vi "H5Sget_simple_extent_dims.vi"(6 "error in (no error)":errorcluster, 9 "HDF5 Space Ref":T1) -> (0 "error out":errorcluster, 1 "Max Dims":u64[](array[numeric]), 2 "Dims":u64[](array[numeric]), 3 "HDF5 Ref out":T1)   [LabVIEW 2017]
doc: "Retrieves dataspace dimension size and maximum size."
uses:
  <vilib>/UPVI/lvhdf5/library.llb/HDF5 Ref.ctl
  <vilib>/UPVI/lvhdf5/hdf5.dll
panel:
  # "LVHDF5 Toolkit\nCopyright (c) 2005-2013 by Jason D. Sommerville\nCopyright (c) 2014 by UPVI, LLC.\n\nThis use and distribution of this file is governed by the terms found in \nLICENSE.txt distributed with this toolkit and installed at\n <user.lib>\\_lvhdf5\\LICENSE.txt"
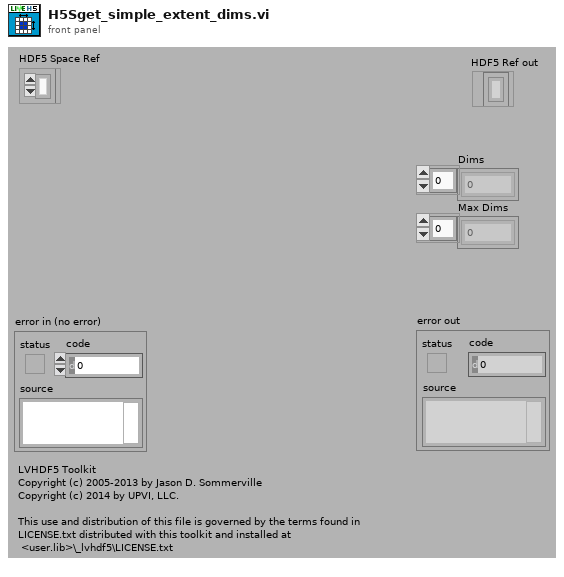
[diagram p1: front panel]
types:
  T1 = typedef "HDF5 Ref.ctl" = refnum<k1>
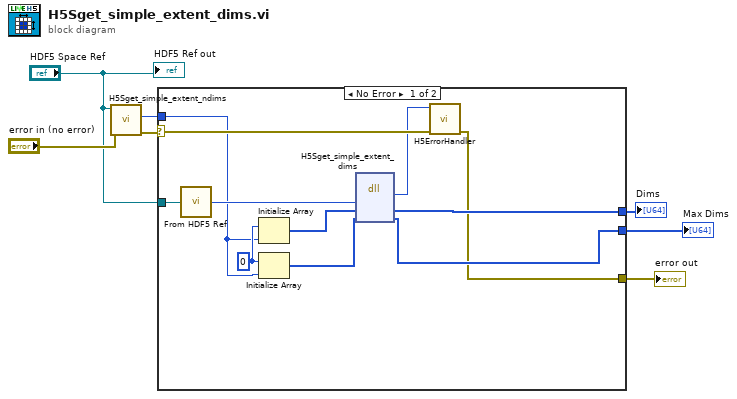
[diagram p0: block diagram]
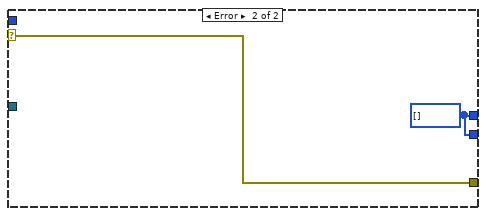
[diagram p2: hidden frame]
diagram:
  n1 = call <vilib>:"H5Sget_simple_extent_ndims.vi"("error in (no error)"="error in (no error)", "HDF5 Space Ref"="HDF5 Space Ref") -> ("error out"=w5:errorcluster, "Rank"=w3:i32)  [unwired: 5 in, 1 out]
  n2 = case shown="No Error" w5 {
    selector: w5 -> [w18 w20]
    tunnel: [w8 w20] -> w7
    tunnel: "HDF5 Space Ref" -> [w17 _]
    tunnel: w3 -> [w13 _]
    tunnel: [w9 w19] -> w2
    tunnel: [w10 w19] -> w1
    frame No Error {
      w14 = u64 0 ("element")
      n3 = call <vilib>:"From HDF5 Ref.vi"("HDF5 Ref"=w17) -> ("I32"=w16:i32)
      n4 = Initialize Array(w14, w13) -> (w11:u64[])
      n5 = Initialize Array(w14, w13) -> (w12:u64[])
      n6 = dll-call lib="C:/Program Files/National Instruments/LabVIEW 2017/vi.lib/UPVI/lvhdf5/hdf5.dll" fn="H5Sget_simple_extent_dims"("space_id"=w16, "dims"=w11, "maxdims"=w12) -> ("return type"=w15:i32, "dims"=w10:u64[], "maxdims"=w9:u64[])  [unwired: 4 in, 2 out]
      n7 = call <vilib>:"H5ErrorHandler.vi"("error in (no error)"=w18, "herr_t"=w15) -> ("error out"=w8:errorcluster)  [unwired: 3 in, 4 out]
    }
    frame Error {
      w19 = i32[] [] ("I32")
    }
  }
  "error out" <- w7
  "Max Dims" <- w2
  "Dims" <- w1
  "HDF5 Ref out" <- "HDF5 Space Ref"
